vi "bin to dec.vi"() -> ()   [LabVIEW 2018]
panel:
  out "Numeric 4":dbl
  in  "Numeric 3":i64 format="%b"
  out "Numeric 2":dbl
  in  "Numeric":dbl
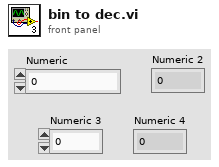
[diagram p1: front panel]
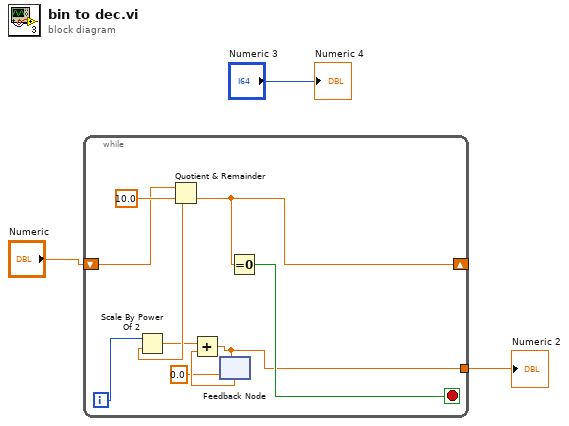
[diagram p0: block diagram]
diagram:
  n1 = while {
    shift-right: [w10] -> _
    shift-left: "Numeric" -> [w11]
    tunnel: [w4] -> w2
    i -> [w9]
    stop <- w12 stop-if-true
    n2 = Quotient & Remainder(x=w11, y=10.0) -> (x-y*floor(x/y)=w8:dbl, floor(x/y)=w10:dbl)
    n3 = Scale By Power Of 2(n=w9, x=w8) -> (x*2^n=w7:dbl)
    n4 = feedback #1(0.0) -> (w6:dbl)
    n5 = Add(x=w7, y=w6) -> (x+y=w4:dbl)
    n6 = feedback-in #1(w4) -> ()
    n7 = Equal To 0?(x=w10) -> (x = 0?=w12:bool)
  }
  "Numeric 2" <- w2
  "Numeric 4" <- "Numeric 3"
